vi "State Machine VI Server.vi"() -> ()   [LabVIEW 2014]
uses:
  Ex 1/Enum.ctl
panel:
  in  "Allow tamperency?":bool=TRUE
  in  "Centered":bool
  in  "Transparancy(%)":dbl(slide) scale=10.0..50.0
  out "?":bool
  in  "STOP":bool
  in  "Executer le processus 2":bool
  in  "Executer le processus 1":bool
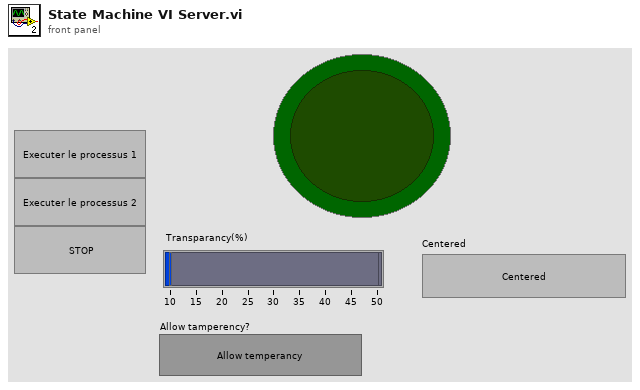
[diagram p1: front panel]
types:
  T1 = enum16{"open", "replace", "create", "open or create", "replace or create", "replace or create with confirmation"}
  T2 = typedef "Enum.ctl" = enum16{"Inactif", "Processus 1", "Processus 2", "Arret"}
  T3 = cluster{"Allow tamperency?":bool, "Transparancy(%)":dbl, "Centered":bool}
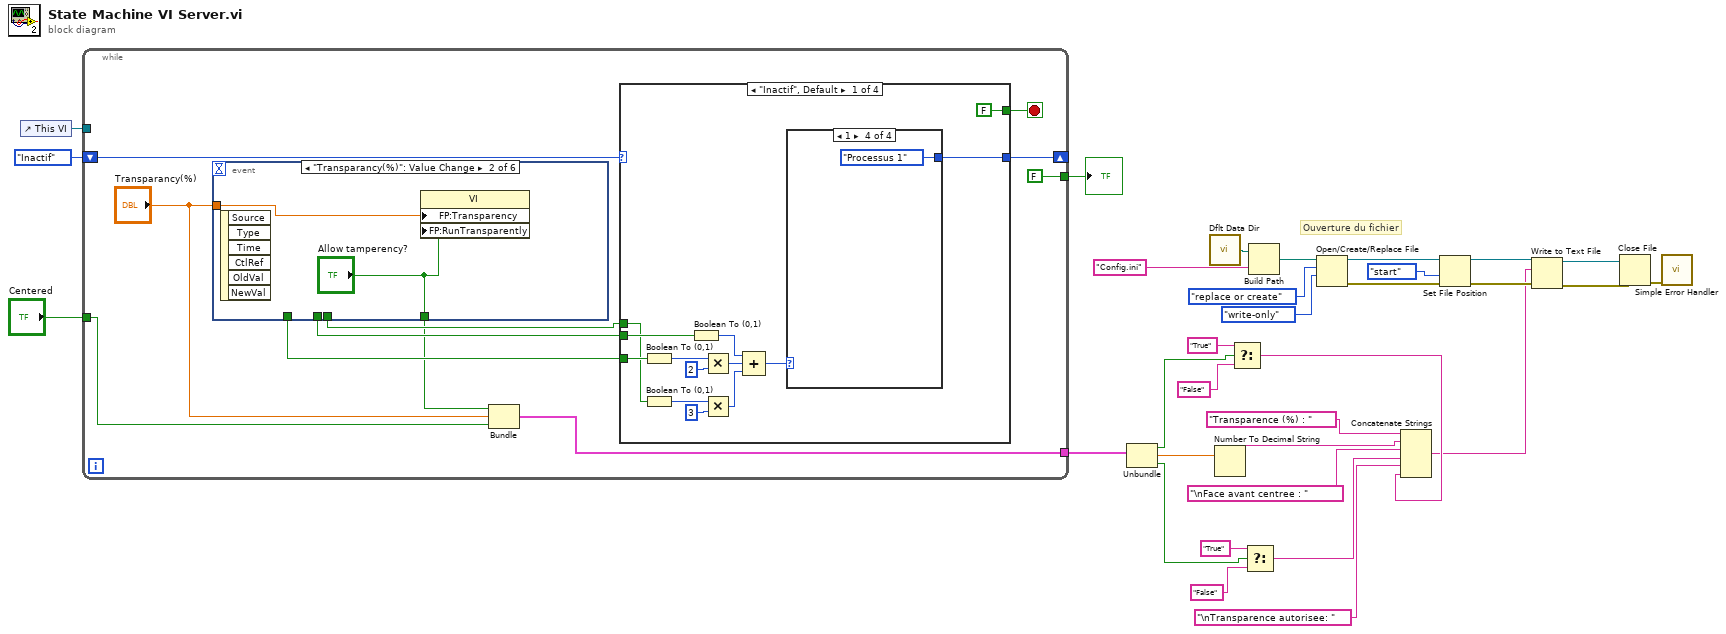
[diagram p0: block diagram]
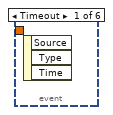
[diagram p2: hidden frame]
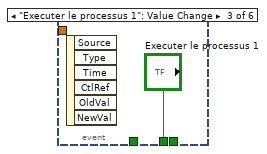
[diagram p3: hidden frame]
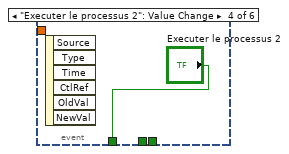
[diagram p4: hidden frame]
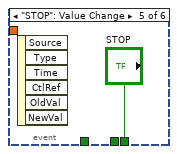
[diagram p5: hidden frame]
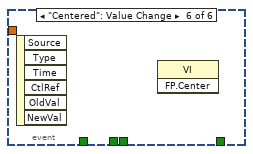
[diagram p6: hidden frame]
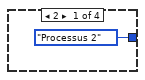
[diagram p7: hidden frame]
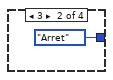
[diagram p8: hidden frame]
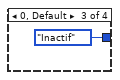
[diagram p9: hidden frame]
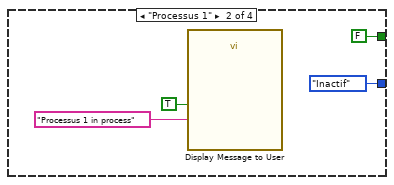
[diagram p10: hidden frame]
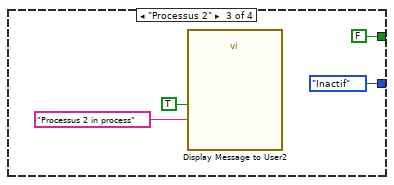
[diagram p11: hidden frame]
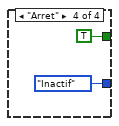
[diagram p12: hidden frame]
diagram:
  # "Ouverture du fichier"
  n1 = control-ref of="This VI"() -> (w30:refnum<vi>)
  n2 = while {
    shift-right: [w42] -> _
    shift-left: Enum."Inactif" -> [w43]
    tunnel: [FALSE] -> w31
    tunnel: w30 -> [_]
    tunnel: "Centered" -> [w34]
    tunnel: [w33] -> w20
    stop <- w41 stop-if-true
    n3 = event shown="[1] \"Transparancy(%)\": Value Change" {
      selector: _ -> [_ _ _ _ _ _]
      dyn-events: _ -> [_ _ _ _ _ _]
      timeout: _ -> [_ _ _ _ _ _]
      tunnel: "Transparancy(%)" -> [_ w45 _ _ _ _]
      tunnel: [_ _ "Executer le processus 1" _ _ _] -> w39
      tunnel: [_ _ _ "Executer le processus 2" _ _] -> w38
      tunnel: [_ _ _ _ "STOP" _] -> w37
      tunnel: [_ "Allow tamperency?" _ _ _ _] -> w36
      event Timeout {
        n4 = event-data() -> ()  [unwired: 1 in, 3 out]
      }
      event "Transparancy(%)": Value Change {
        n5 = event-data() -> ()  [unwired: 1 in, 6 out]
        n6 = property class="VI"("FP:Transparency"=w45, "FP:RunTransparently"="Allow tamperency?") -> ()  [unwired: 2 in, 2 out]
      }
      event "Executer le processus 1": Value Change {
        n7 = event-data() -> ()  [unwired: 1 in, 6 out]
      }
      event "Executer le processus 2": Value Change {
        n8 = event-data() -> ()  [unwired: 1 in, 6 out]
      }
      event "STOP": Value Change {
        n9 = event-data() -> ()  [unwired: 1 in, 6 out]
      }
      event "Centered": Value Change {
        n10 = event-data() -> ()  [unwired: 1 in, 6 out]
        n11 = invoke class="VI" method="FP.Center"() -> ()  [unwired: 3 in, 3 out]
      }
    }
    n12 = Bundle("Allow tamperency?"=w36, "Transparancy(%)"="Transparancy(%)", "Centered"=w34) -> (w33:T3)  [unwired: 1 in]
    n13 = case shown="\"Inactif\", Default" w43 {
      tunnel: [w53 Enum."Inactif" Enum."Inactif" Enum."Inactif"] -> w42
      tunnel: [FALSE FALSE FALSE TRUE] -> w41
      tunnel: w39 -> [w51 _ _ _]
      tunnel: w38 -> [w50 _ _ _]
      tunnel: w37 -> [w49 _ _ _]
      frame "Inactif", Default {
        n14 = Boolean To (0,1)(Boolean=w50) -> (0, 1=w61:i16)
        n15 = Boolean To (0,1)(Boolean=w49) -> (0, 1=w60:i16)
        n16 = Boolean To (0,1)(Boolean=w51) -> (0, 1=w59:i16)
        n17 = Multiply(x=w61, y=2) -> (x*y=w58:i32)
        n18 = Multiply(x=w60, y=3) -> (x*y=w54:i32)
        n19 = Compound Arithmetic op=ADD(w59, w58, w54) -> (w55:i32)
        n20 = case shown="1" w55 {
          tunnel: [Enum."Processus 2" Enum."Arret" Enum."Inactif" Enum."Processus 1"] -> w53
          frame 2 {
          }
          frame 3 {
          }
          frame 0, Default {
          }
          frame 1 {
          }
        }
      }
      frame "Processus 1" {
        n21 = call "Display Message to User"("Enable"=TRUE, "Message"="Processus 1 in process" ("message")) -> ()  [unwired: 8 in, 2 out]
      }
      frame "Processus 2" {
        n22 = call "Display Message to User2"("Enable"=TRUE, "Message"="Processus 2 in process" ("message")) -> ()  [unwired: 8 in, 2 out]
      }
      frame "Arret" {
      }
    }
  }
  "?" <- w31
  n23 = Unbundle(w20) -> ("Allow tamperency?"=w9:bool, "Transparancy(%)"=w18:dbl, "Centered"=w13:bool)
  n24 = call <vilib>:"Dflt Data Dir.vi"() -> ("App:Default Data Directory"=w25:path)
  n25 = Number To Decimal String(number=w18) -> (decimal integer string=w17:string)  [unwired: 1 in]
  n26 = Select(t="True", s=w9, f="False" ("t")) -> (s? t:f=w8:string)
  n27 = Select(t="True", s=w13, f="False" ("t")) -> (s? t:f=w12:string)
  n28 = Build Path(base path=w25, name or relative path="Config.ini" ("Nom de fichier")) -> (appended path=w22:path)
  n29 = Open/Create/Replace File(file path (use dialog)=w22, operation (0:open)=T1."replace or create", access (0:read/write)=enum16{"read/write", "read-only", "write-only"}."write-only") -> (refnum out=w28:refnum<file>, error out=w27:errorcluster)  [unwired: 1 in, 3 out]
  n30 = Concatenate Strings("Transparence (%) : " ("string"), w17, "\nFace avant centree : " ("string"), w12, "\nTransparence autorisee: " ("string"), w8) -> (w5:string)
  n31 = Set File Position(refnum=w28, from (0:start)=enum16{"start", "end", "current"}."start", error in=w27) -> (refnum out=w4:refnum<file>, error out=w6:errorcluster)  [unwired: 1 in]
  n32 = Write to Text File(file (use dialog)=w4, text=w5, error in=w6) -> (refnum out=w3:refnum<file>, error out=w2:errorcluster)  [unwired: 1 in, 1 out]
  n33 = Close File(refnum=w3, error in=w2) -> (error out=w7:errorcluster)  [unwired: 1 out]
  n34 = call <vilib>:"Simple Error Handler.vi"("error in (no error)"=w7) -> ()  [unwired: 4 in, 5 out]
